vi "DSF.Engine.Pool.Destroy FIFO.vi"(8 "error in (no error)":errorcluster, 11 "Pool in":refnum<class "DSF.Engine.Pool.lvclass">) -> (0 "error out":errorcluster, 3 "Pool out":refnum<class "DSF.Engine.Pool.lvclass">)   [LabVIEW 2017, in "Data Sharing Framework Engine.lvlib" / "DSF.Engine.Pool.lvclass"]
uses:
  DSF.Engine.Pool.lvclass
  DSF.Engine.Pool.lvclass/DSF.Engine.Pool.ctl
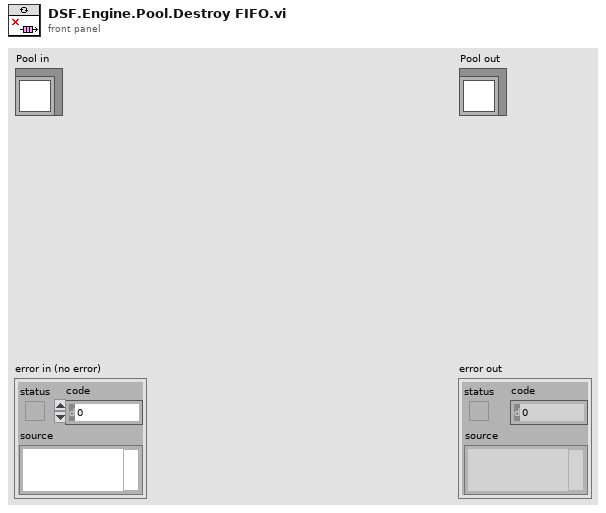
[diagram p1: front panel]
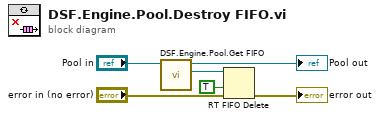
[diagram p0: block diagram]
diagram:
  n1 = call "DSF.Engine.Pool.Get FIFO.vi"("Pool in"="Pool in") -> ("FIFO"=w2:refnum<k33>, "Pool out"=→"Pool out":refnum<class "DSF.Engine.Pool.lvclass">)  [unwired: 9 in]
  n2 = RT FIFO Delete(0:w2, 2:TRUE ("force destroy? (F)"), 3:"error in (no error)") -> (11:→"error out":errorcluster)
